vi "EQE_SystemSetup_HZ.vi"(2 "CFG File Path":string, 3 "ATR File Path":string) -> (0 "Error":string, 1 "Error Code":i32)   [LabVIEW 2017]
uses:
  Program Files (x86)/Bentham/SDK/code examples/LabView/8.0/BenHw/benhw32_stdcall.dll
panel:
  out "Initialise System":i32
  out "Load Setup":i32
  out "Build System Model":i32
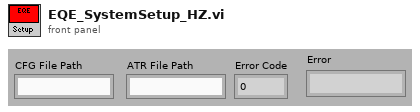
[diagram p1: front panel]
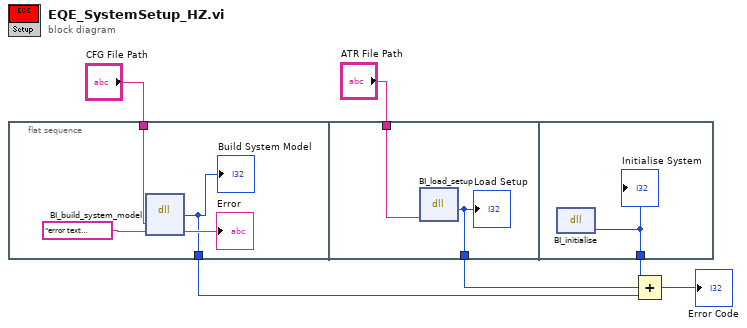
[diagram p0: block diagram]
diagram:
  n1 = flat-sequence {
    tunnel: "CFG File Path" -> [w8]
    tunnel: [w7] -> w2
    tunnel: "ATR File Path" -> [w12]
    tunnel: [w11] -> w3
    tunnel: [w13] -> w4
    frame #0 {
      n2 = dll-call lib="C:/Program Files (x86)/Bentham/SDK/code examples/LabView/8.0/BenHw/benhw32_stdcall.dll" fn="BI_build_system_model"("cfgfile"=w8, "error"="error text                                       with lots of extra characters for reallly long reports ") -> ("return type"=w7:i32, "error"=→"Error":string)  [unwired: 4 in, 2 out]
      "Build System Model" <- w7
    }
    frame #1 {
      n3 = dll-call lib="C:/Program Files (x86)/Bentham/SDK/code examples/LabView/8.0/BenHw/benhw32_stdcall.dll" fn="BI_load_setup"("atr_file"=w12) -> ("return type"=w11:i16)  [unwired: 4 in, 2 out]
      "Load Setup" <- w11
    }
    frame #2 {
      n4 = dll-call lib="C:/Program Files (x86)/Bentham/SDK/code examples/LabView/8.0/BenHw/benhw32_stdcall.dll" fn="BI_initialise"() -> ("return type"=w13:i16)  [unwired: 3 in, 2 out]
      "Initialise System" <- w13
    }
  }
  n5 = Compound Arithmetic op=ADD(w4, w3, w2) -> (→"Error Code":i32)
